vi "Initialize.vi"(8 "error in (no error)":errorcluster, 10 "Angle-Value Pairs":T1[](array[typedef]), 11 "LinearInterpolation in":refnum<class "LinearInterpolation.lvclass">) -> (0 "error out":errorcluster, 3 "LinearInterpolation out":refnum<class "LinearInterpolation.lvclass">)   [LabVIEW 2012, in "LinearInterpolation.lvclass"]
doc: "For a given array of angle-value pairs, it sorts the angles in ascending order and saves them as instance variables in the object. \n\nNote: the calculate function will not work unless the angles are sorted in this way"
uses:
  LinearInterpolation.lvclass
  AngleValuePair.ctl
  LinearInterpolation.lvclass/LinearInterpolation.ctl
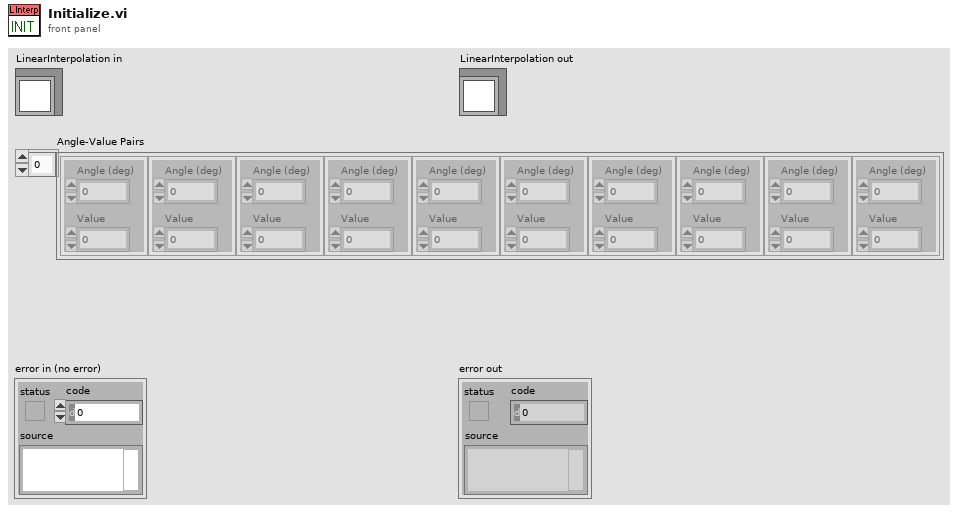
[diagram p1: front panel]
types:
  T1 = typedef "AngleValuePair.ctl" = cluster{"Angle (deg)":dbl, "Value":dbl}
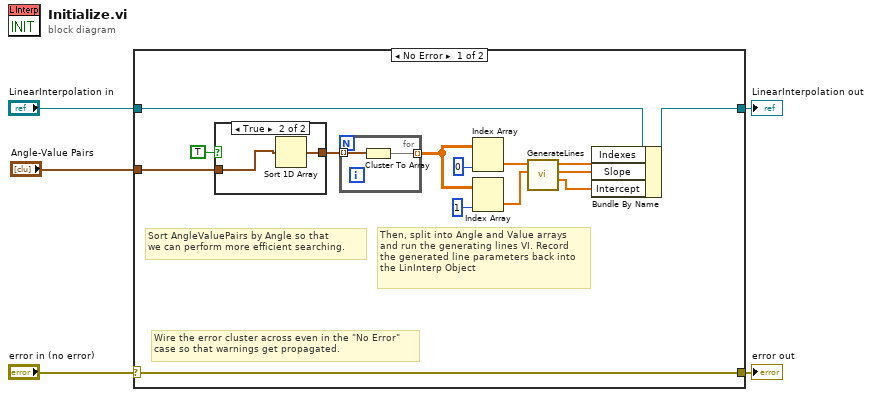
[diagram p0: block diagram]
diagram:
  n1 = case shown="No Error" "error in (no error)" {
    selector: "error in (no error)" -> [w19 w26]
    tunnel: [w19 w26] -> w4
    tunnel: [w13 w25] -> w2
    tunnel: "LinearInterpolation in" -> [w14 w25]
    tunnel: "Angle-Value Pairs" -> [w12 _]
    frame No Error {
      # "Sort AngleValuePairs by Angle so that \nwe can perform more efficient searching."
      # "Then, split into Angle and Value arrays \nand run the generating lines VI. Record\nthe generated line parameters back into\nthe LinInterp Object"
      # "Wire the error cluster across even in the \"No Error\"\ncase so that warnings get propagated."
      n2 = case shown="True" TRUE {
        tunnel: [w20 w22] -> w18
        tunnel: w12 -> [w20 w21]
        frame False {
        }
        frame True {
          n3 = Sort 1D Array(array=w21) -> (sorted array=w22:T1[])
        }
      }
      n4 = for {
        tunnel: w18 -> [w23] mode=indexing
        tunnel: [w24] -> w15 mode=indexing
        n5 = Cluster To Array(cluster=w23) -> (array=w24:dbl[])
      }
      n6 = Index Array(array=w15, index (col)=0) -> (element=w10:dbl[])  [unwired: 1 in]
      n7 = Index Array(array=w15, index (col)=1) -> (element=w9:dbl[])  [unwired: 1 in]
      n8 = call "GenerateLines.vi"("Values"=w9, "Angles"=w10) -> ("Intercept"=w6:dbl[], "Slope"=w7:dbl[], "Angles/Indicies"=w8:dbl[])  [unwired: 7 in]
      n9 = Bundle By Name(cluster=w14, "Indexes"=w8, "Slope"=w7, "Intercept"=w6) -> (w13:refnum<class "LinearInterpolation.lvclass">)
    }
    frame Error {
    }
  }
  "error out" <- w4
  "LinearInterpolation out" <- w2
